vi "EjemplousandoFor.vi"() -> ()   [LabVIEW 2022 SP3]
panel:
  out "Numeric":i32
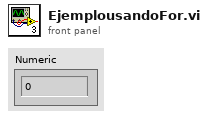
[diagram p1: front panel]
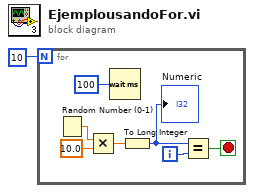
[diagram p0: block diagram]
diagram:
  n1 = for {
    N: 10 -> [_]
    i -> [w4]
    stop <- w3 stop-if-true
    n2 = Random Number (0-1)() -> (number: 0 to 1=w8:dbl)
    n3 = Multiply(x=w8, y=10.0) -> (x*y=w5:dbl)
    n4 = Wait (ms)(milliseconds to wait=u32 100) -> ()  [unwired: 1 out]
    n5 = To Long Integer(number=w5) -> (32bit integer=w2:i32)
    "Numeric" <- w2
    n6 = Equal?(x=w2, y=w4) -> (x = y?=w3:bool)
  }
